vi "LaserMaster.vi"() -> ()   [LabVIEW 2014]
uses:
  Serial/Serial.lvclass
  <vilib>/Utility/file.llb/Write To Spreadsheet File (string).vi
panel:
  out "Discovery?":bool
  out "Humidity Threshold":dbl
  in  "Power (mW) 2":dbl format="%#.0f"
  out "SavePath":path
  out "Start time":timestamp
  out "Step":dbl
  out "State next step":string
  in  "stop":bool
  out "Query backup List":string[][](array[string])=[["?L", " 0\r"], ["?K", " 0\r"], ["?F", " 0\r"], ["?FH", " 2\r"], ["?SHUTTER", " 0\r"], ["?UF", " 0\r"], ["?PHLDC", " 1\r"], ["?PZTMC", " 0\r"], ["?PZTXC", " 2.24\r"], ["?PZTYC", " 2.14\r"], ["?PHLDP", " 0\r"], ["?PZTMP", " 0\r"], ["?PZTXP", " 2.58\r"], ["?PXTYP", "  Query Error:?PXTYP\r"], ["?PTRK", "  Query Error:?PTRK\r"], ["?MDLK", " 0\r"], ["?PP", " 0.80\r"], ["?TS", " 0\r"], ["?SM", " 1\r"], ["?HM", " 1\r"], ["?VW", " 850\r"], ["?STPRPOS", " 2096\r"], ["?C", " 0.00\r"], ["?D1C", " 0.08\r"], ["?D2C", " -0.43\r"], ["?BT", " 20.07\r"], ["?D1T", " 24.20\r"], ["?D2T", " 24.20\r"], ["?VT", " 20.72\r"], ["?LBOT", " 148.45\r"], ["?ET", " 39.01\r"], ["?D1ST", " 24.20\r"], ["?D2ST", " 24.20\r"], ["?VST", " 30.00\r"], ["?LBOST", " 148.41\r"], ["?EST", " 39.00\r"], ["?D1TD", " 500.12\r"], ["?D2TD", " 464.53\r"], ["?VD", " 0.00\r"], ["?LBOD", " 5358.08\r"], ["?ED", " 2152.46\r"], ["?D1HST", " 21.35\r"], ["?D2HST", " 21.48\r"], ["?LBOH", " 1\r"], ["?LRS", " 2\r"], ["?D1SS", " 1\r"], ["?D2SS", " 1\r"], ["?VSS", " 0\r"], ["?LBOSS", " 1\r"], ["?ESS", " 1\r"], ["?D1H", "  351.54\r"], ["?D2H", "  351.52\r"], ["?HH", " 37\r"], ["?D1V", " 0.19\r"], ["?D2V", " 0.18\r"], ["?SV", " 8.26,8.26,9.57\r"], ["?MB", "  Query Error:?MB\r"], ["?PI", " 2BC\r"], ["?BV", " 13.24\r"], ["?AMDLK", " 1\r"], ["?PZTS", "  Query Error:?PZTS\r"], ["?TMAX", " 1080\r"], ["?TMIN", " 680\r"], ["?ALIGN", " 0\r"], ["?ALIGNP", " 250\r"], ["?ALIGNW", " 730\r"], ["?LFP", " 0\r"], ["?PZTXCM", " 8.11\r"], ["?PZTXCP", " -10.30\r"], ["?PZTXPM", " 8.11\r"], ["?PZTXPP", " 3.06\r"], ["?PZTYCM", " 8.11\r"], ["?PZTYCP", " -14.28\r"], ["?PZTYPM", " 8.11\r"], ["?PZTYPP", " 11.74\r"], ["?RH", " 0\r"], ["?SN", " 9571\r"], ["?ST", " Standby\r"], ["?GDDCURVE", " 0\r"], ["?GDD", " 0\r"], ["?GDDCURVEN", " ZERO\r"], ["?CURVEN", " OUT OF RANGE\r"], ["?COMP", " 1\r"], ["?HMCOMP", " 1\r"], ["?GDDMAX", " 17333\r"], ["?GDDMIN", "0"]]
  out "Laser Info":i32
  out "Shutter off time":dbl
  out "Quiting":dbl
  out "Backuper state":string
  in  "Tab Control":T1(tab)
  out "Power 2":i32
  in  "Align 2":bool
  in  "Shutter 2":bool
  in  "Lock":bool
  in  "Auto":bool
  out "Baseplate Temp (C)":dbl(slide) scale=20.0..40.0
  in  "Dither hold":bool
  in  "Shutter":bool
  out "Laser Status":bool
  out "Power (mW)":dbl(knob) scale=0.0..5000.0
  out "Walking":bool
  out "Sleeping":bool
  out "ModeLocked":bool
  out "Backing up":bool
  in  "Wavelength":dbl=920.0
  in  "GDD":dbl
  in  "QUIT":bool
  out "Max":string
  in  "Align":bool
  in  "Def. Wavelength":dbl=920.0
  in  "Dither auto":dbl=120.0
  in  "Dither timer":dbl=5.0
  out "Faults":string
  in  "Home motor":bool
  in  "Optimize":bool
  in  "WV Walk":bool
  in  "Standby Time (min)":dbl=120.0
  in  "Sleep":bool
  in  "Backup":bool
  in  "Auto-Backup \nIdle Time (min)":dbl=30.0
  out "Operating Status":string
  out "Tunning Status":i32
  out "Idle Time":dbl format="%.1f"
  out "Laser On Time":dbl format="%#.1f"
  in  "Laser Control":bool
  in  "Command Line":string
  out "Laser Response":string
  in  "Refresh":bool
  out "Query List":string[][](array[string])
  out "queue #":i32
  # "LASER"
  # "LASER fine-tune"
  # "BACKUP"
  # "Timers"
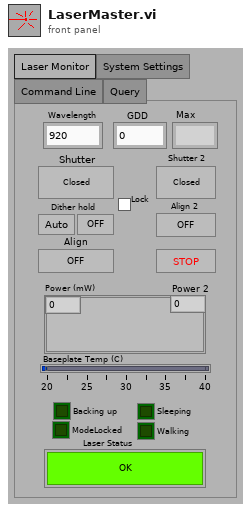
[diagram p1: front panel]
types:
  T1 = enum32{"Laser Monitor", "System Settings", "Command Line", "Query"}
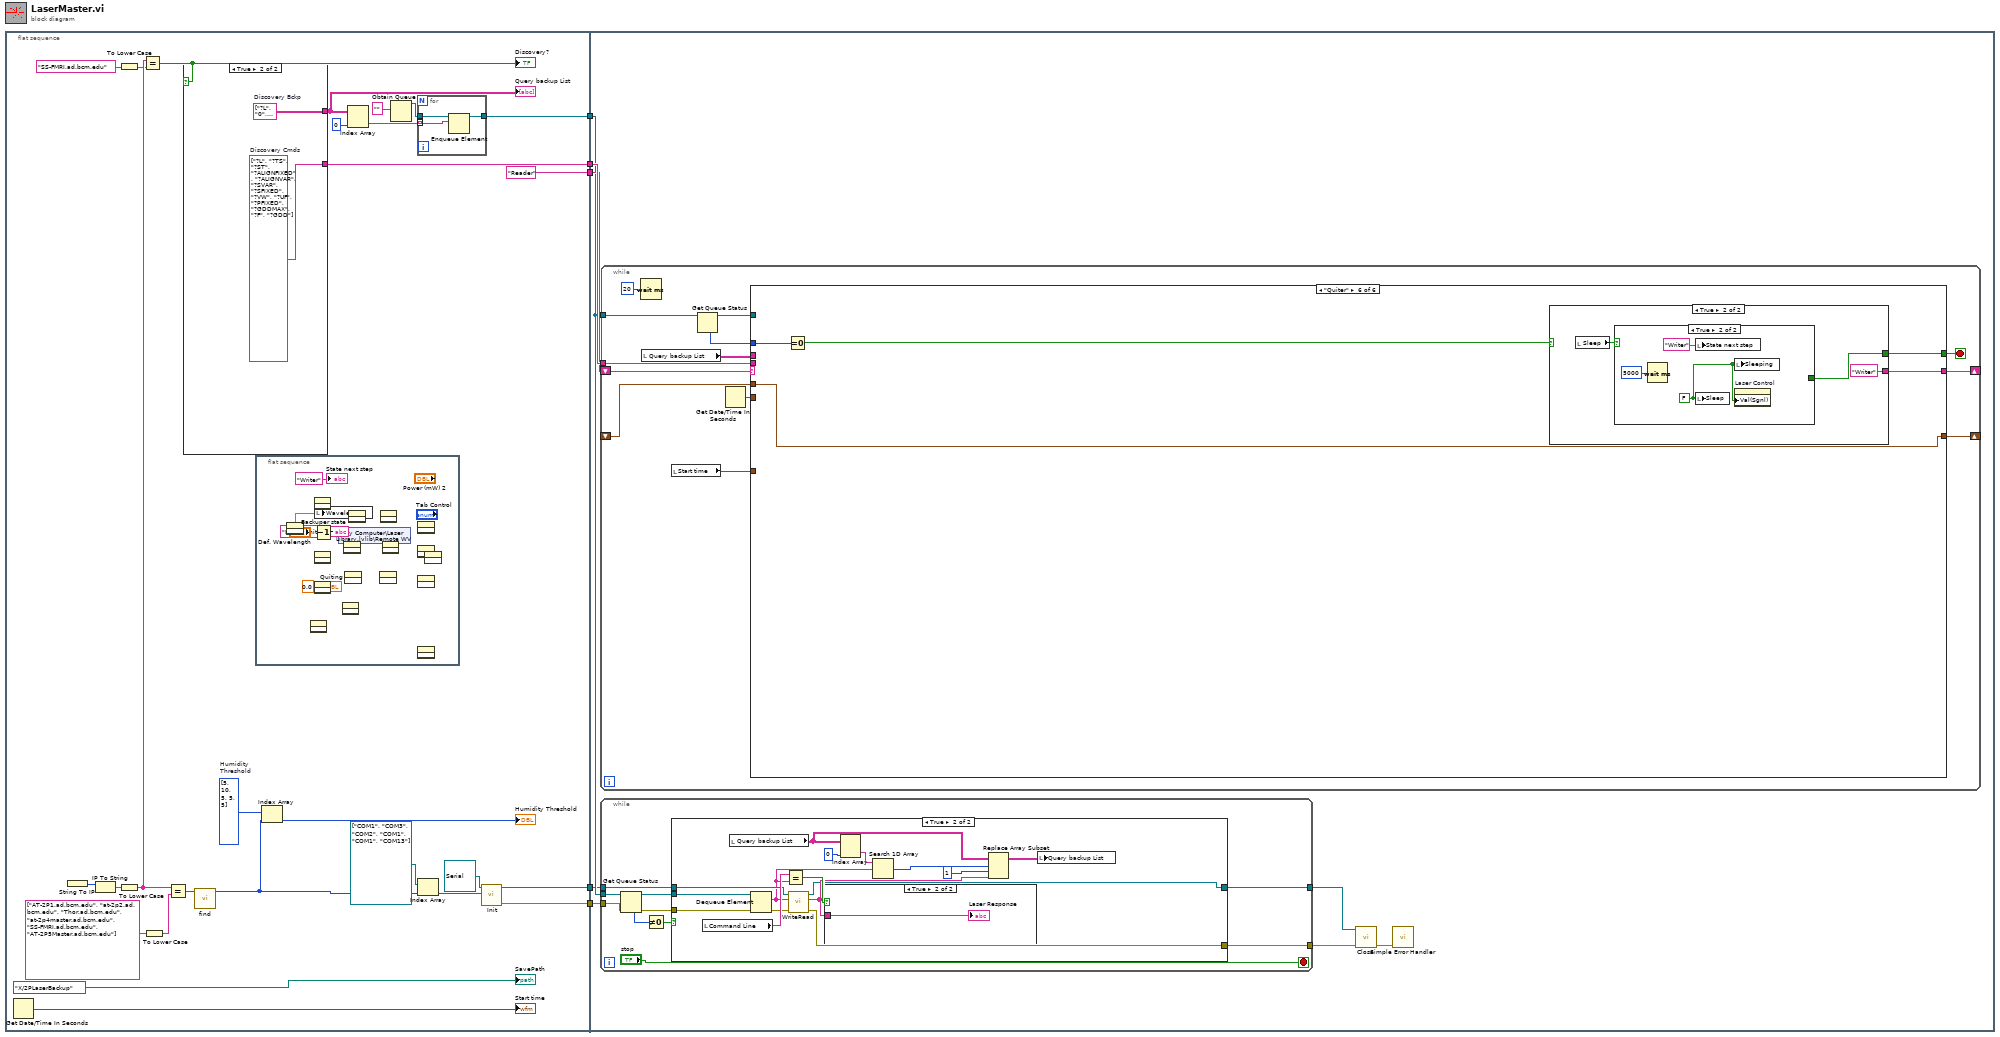
[diagram p0: block diagram]
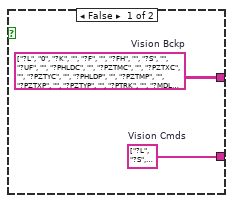
[diagram p2: hidden frame]
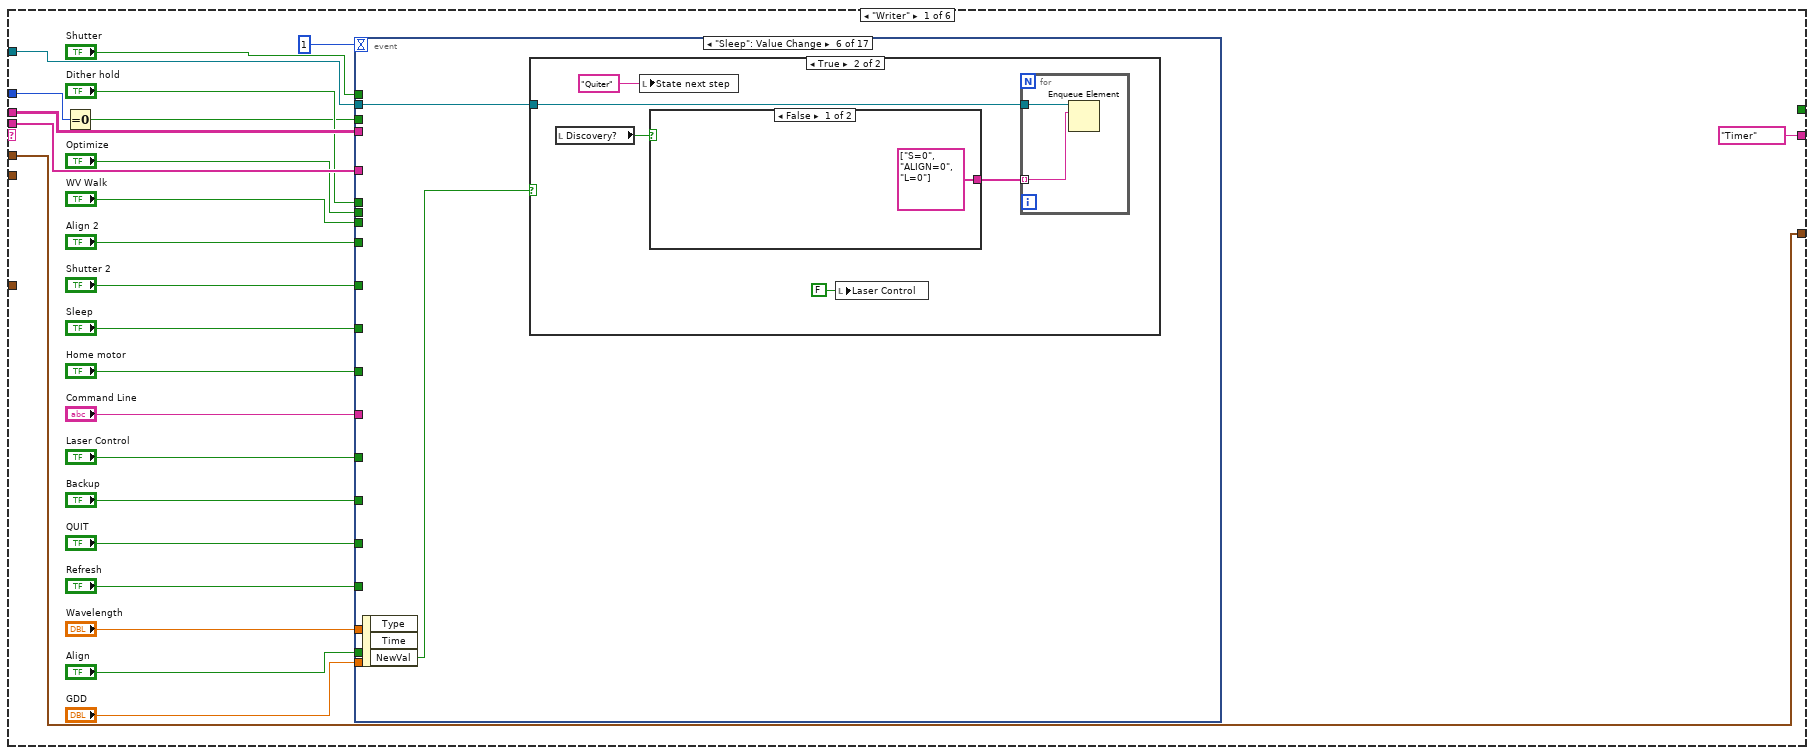
[diagram p5: hidden frame]
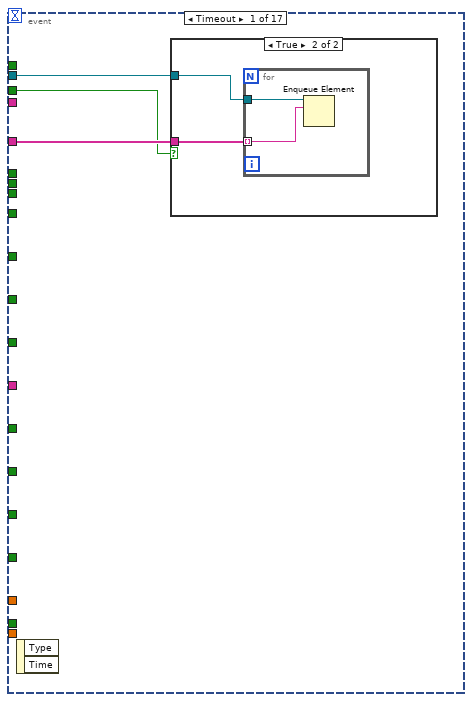
[diagram p6: hidden frame]
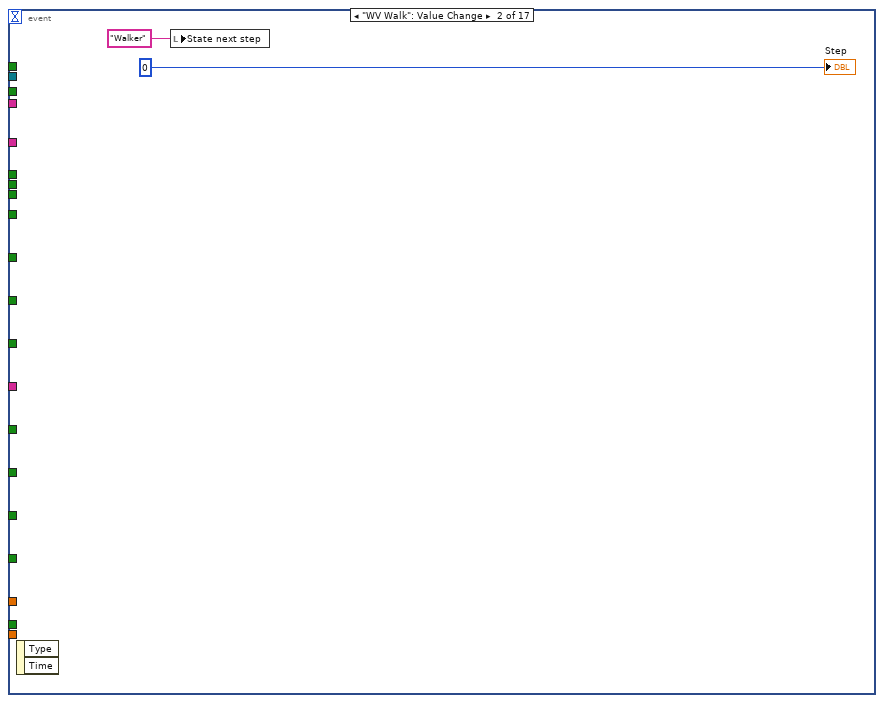
[diagram p8: hidden frame]
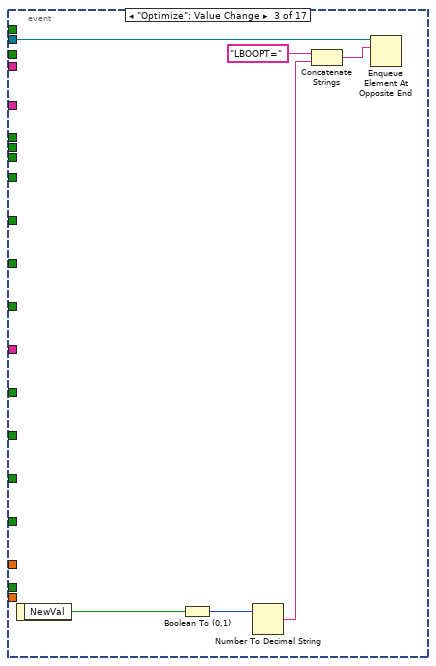
[diagram p9: hidden frame]
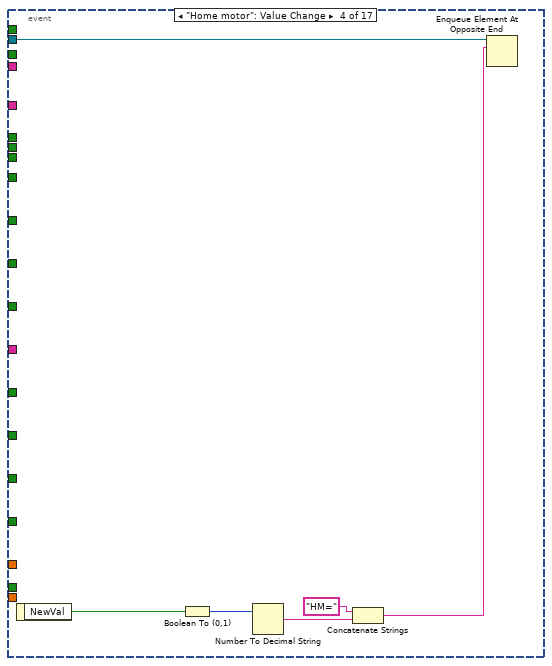
[diagram p10: hidden frame]
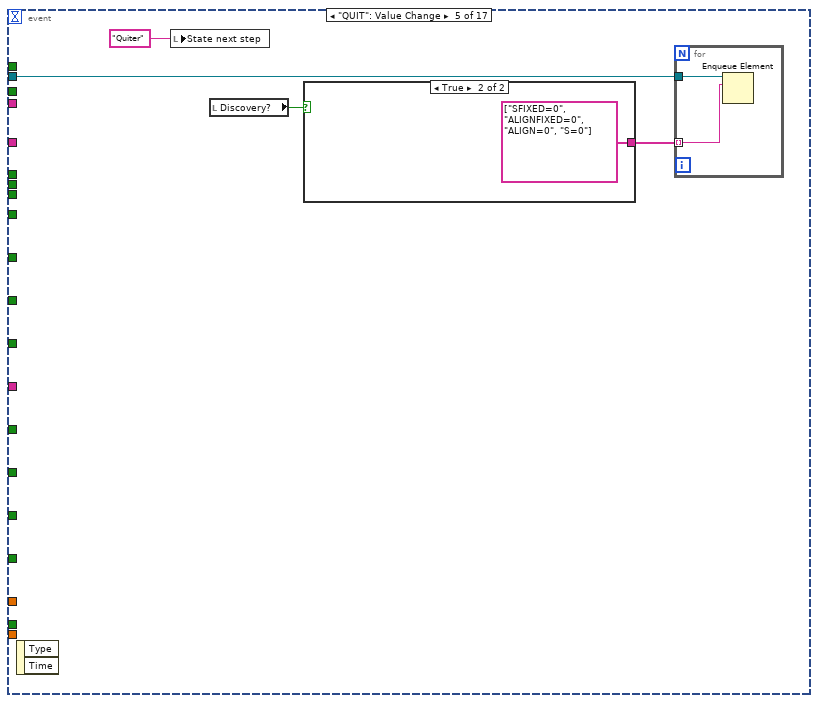
[diagram p11: hidden frame]
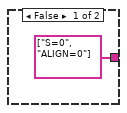
[diagram p12: hidden frame]
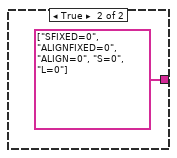
[diagram p14: hidden frame]
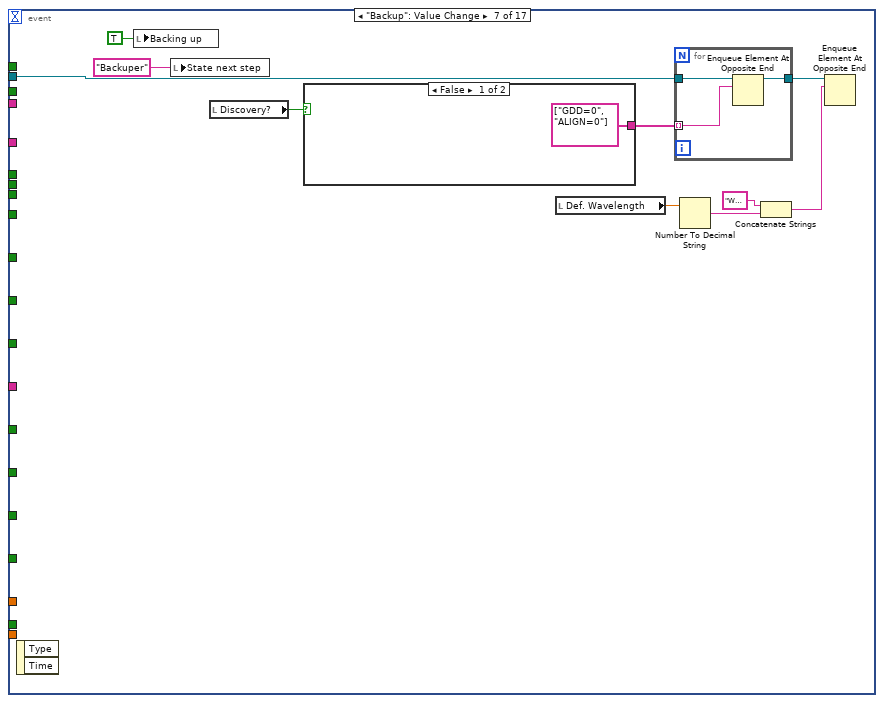
[diagram p15: hidden frame]
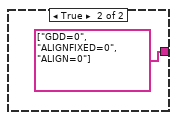
[diagram p16: hidden frame]
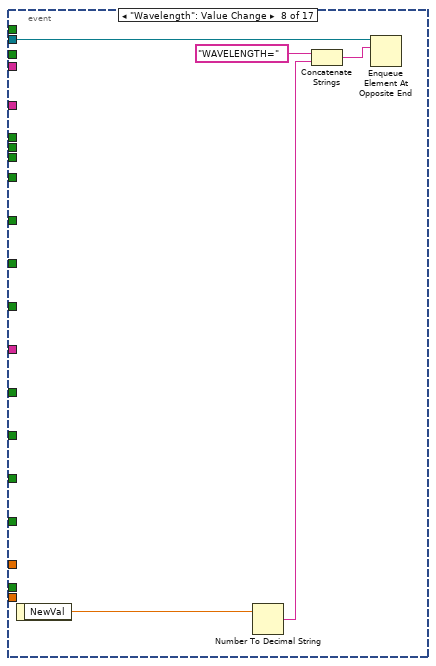
[diagram p17: hidden frame]
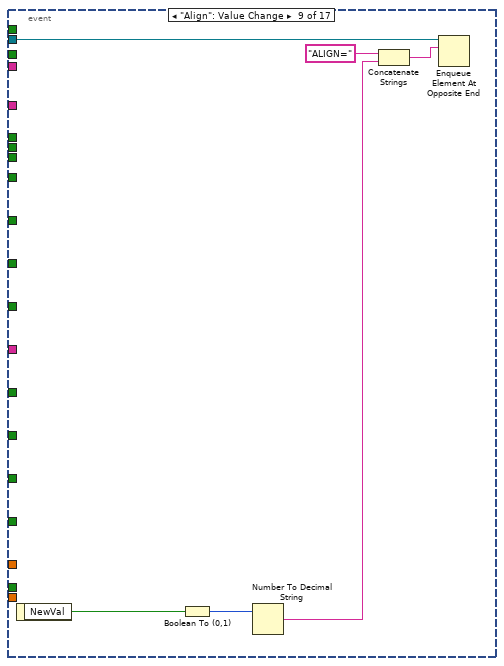
[diagram p18: hidden frame]
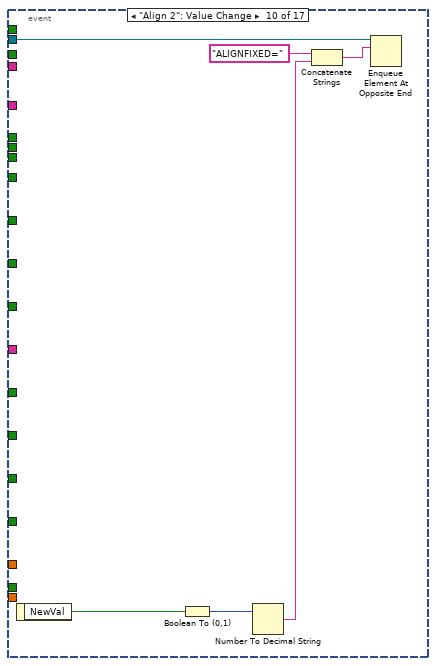
[diagram p19: hidden frame]
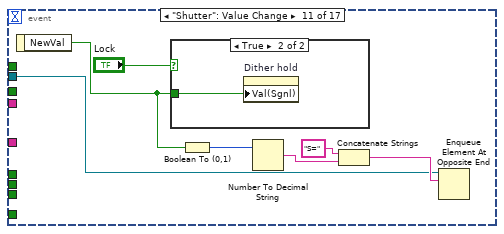
[diagram p20: hidden frame]
diagram:
  n1 = flat-sequence {
    tunnel: [w27] -> w5
    tunnel: [w10] -> w4
    tunnel: ["Reader"] -> w3
    tunnel: [w7] -> w2
    tunnel: [w6] -> w1
    tunnel: w5 -> [w50]
    tunnel: w4 -> [w52]
    tunnel: w3 -> [w51]
    tunnel: w2 -> [w49]
    tunnel: w1 -> [w48]
    frame #0 {
      w19 = i32[] [5, 10, 5, 5, 5]  # Humidity  Threshold
      n2 = Get Date/Time In Seconds() -> (seconds since 1Jan1904=→"Start time":timestamp)
      n3 = String To IP() -> (0:w24:u32)  [unwired: 1 in]
      n4 = IP To String(2:w24) -> (0:w22:string)  [unwired: 1 in]
      n5 = To Lower Case(string="SS-FMRI.ad.bcm.edu") -> (all lower case string=w13:string)
      n6 = To Lower Case(string=w22) -> (all lower case string=w15:string)
      n7 = Equal?(x=w15, y=w13) -> (x = y?=w12:bool)
      "Discovery?" <- w12
      n8 = To Lower Case(string=string[] ["AT-2P1.ad.bcm.edu", "at-2p2.ad.bcm.edu", "Thor.ad.bcm.edu", "at-2p4master.ad.bcm.edu", "SS-FMRI.ad.bcm.edu", "AT-2P5Master.ad.bcm.edu"]) -> (all lower case string=w23:string[])
      n9 = Equal?(x=w15, y=w23) -> (x = y?=w17:bool[])
      n10 = case shown="True" w12 {
        tunnel: [w34 w36] -> w11
        tunnel: [w33 w35] -> w10
        frame False {
          w33 = string[] ["?L", "?S", "?VW", "?ALIGN", "?PHLDP", "?UF", "?GDD", "?TS", "?ST", "?MDLK", "?GDDMAX", "?F", "?RH", "?BT"]  # Vision Cmds
          w34 = string[][] [["?L", "0"], ["?K", ""], ["?F", ""], ["?FH", ""], ["?S", ""], ["?UF", ""], ["?PHLDC", ""], ["?PZTMC", ""], ["?PZTXC", ""], ["?PZTYC", ""], ["?PHLDP", ""], ["?PZTMP", ""], ["?PZTXP", ""], ["?PZTYP", ""], ["?PTRK", ""], ["?MDLK", ""], ["?PP", ""], ["?TS", ""], ["?SM", ""], ["?HM", ""], ["?VW", ""], ["?STPRPOS", ""], ["?C", ""], ["?D1C", ""], ["?D2C", ""], ["?BT", ""], ["?D1T", ""], ["?D2T", ""], ["?VT", ""], ["?LBOT", ""], ["?ET", ""], ["?D1ST", ""], ["?D2ST", ""], ["?VST", ""], ["?LBOST", ""], ["?EST", ""], ["?D1TD", ""], ["?D2TD", ""], ["?VD", ""], ["?LBOD", ""], ["?ED", ""], ["?D1HST", ""], ["?D2HST", ""], ["?LBOH", ""], ["?LRS", ""], ["?D1SS", ""], ["?D2SS", ""], ["?VSS", ""], ["?LBOSS", ""], ["?ESS", ""], ["?D1H", ""], ["?D2H", ""], ["?HH", ""], ["?D1V", ""], ["?D2V", ""], ["?SV", ""], ["?PI", ""], ["?BV", ""], ["?AMDLK", ""], ["?PZTS", ""], ["?TMAX", ""], ["?TMIN", ""], ["?ALIGN", ""], ["?ALIGNP", ""], ["?ALIGNW", ""], ["?LFP", ""], ["?PZTXCM", ""], ["?PZTXCP", ""], ["?PZTXPM", ""], ["?PZTXPP", ""], ["?PZTYCM", ""], ["?PZTYCP", ""], ["?PZTYPM", ""], ["?PZTYPP", ""], ["?RH", ""], ["?SN", ""], ["?ST", ""], ["?GDDCURVE", ""], ["?GDD", ""], ["?GDDCURVEN", ""], ["?COMP", ""], ["?HMCOMP", ""], ["?GDDMAX", ""], ["?GDDMIN", ""]]  # Vision Bckp
        }
        frame True {
          w35 = string[] ["?L", "?TS", "?ST", "?ALIGNFIXED", "?ALIGNVAR", "?SVAR", "?SFIXED", "?VW", "?UF", "?PFIXED", "?GDDMAX", "?F", "?GDD"]  # Discovery Cmds
          w36 = string[][] [["?L", "0"], ["?K", ""], ["?TS", ""], ["?ST", ""], ["?ALIGNFIXED", ""], ["?ALIGNVAR", ""], ["?SVAR", ""], ["?SFIXED", ""], ["?VW", ""], ["?UF", ""], ["?PFIXED", ""], ["?HB", ""], ["?HRB", ""], ["?GDDCURVE", ""], ["?GDDCURVEN", ""], ["?GDD", ""], ["?GDDMAX", ""], ["?GDDMIN", ""], ["?SN", ""], ["?F", ""], ["?FT", ""], ["?FH", ""], ["?FHT", ""]]  # Discovery Bckp
        }
      }
      "Query backup List" <- w11
      n11 = call "find.vi"("Array"=w17) -> ("Index"=w16:i32)  [unwired: 10 in]
      n12 = flat-sequence {
        frame #0 {
          n13 = invoke on="ModeLocked" class="Bool (strict)" method="Reinit To Default"() -> ()  [unwired: 3 in, 3 out]
          n14 = invoke on="Align" class="Bool (strict)" method="Reinit To Default"() -> ()  [unwired: 3 in, 3 out]
          n15 = Decrement(x="Def. Wavelength") -> (x-1=w38:dbl)
          n16 = invoke on="Home motor" class="Bool" method="Reinit To Default"() -> ()  [unwired: 3 in, 3 out]
          n17 = invoke on="stop" class="Bool (strict)" method="Reinit To Default"() -> ()  [unwired: 3 in, 3 out]
          n18 = invoke on="Sleep" class="Bool (strict)" method="Reinit To Default"() -> ()  [unwired: 3 in, 3 out]
          n19 = local write "Wavelength"("Def. Wavelength") -> ()
          n20 = shared-variable "My Computer\\Laser Library.lvlib\\Remote WV"(w38) -> ()  [unwired: 1 in, 1 out]
          n21 = invoke on="WV Walk" class="Bool (strict)" method="Reinit To Default"() -> ()  [unwired: 3 in, 3 out]
          n22 = invoke on="Walking" class="Bool (strict)" method="Reinit To Default"() -> ()  [unwired: 3 in, 3 out]
          n23 = invoke on="Backup" class="Bool (strict)" method="Reinit To Default"() -> ()  [unwired: 3 in, 3 out]
          n24 = invoke on="Auto" class="Bool (strict)" method="Reinit To Default"() -> ()  [unwired: 3 in, 3 out]
          n25 = invoke on="Optimize" class="Bool" method="Reinit To Default"() -> ()  [unwired: 3 in, 3 out]
          n26 = invoke on="Sleeping" class="Bool (strict)" method="Reinit To Default"() -> ()  [unwired: 3 in, 3 out]
          n27 = invoke on="Refresh" class="Bool (strict)" method="Reinit To Default"() -> ()  [unwired: 3 in, 3 out]
          n28 = invoke on="Idle Time" class="DigNum (strict)" method="Reinit To Default"() -> ()  [unwired: 3 in, 3 out]
          n29 = invoke on="Laser Control" class="Bool (strict)" method="Reinit To Default"() -> ()  [unwired: 3 in, 3 out]
          n30 = invoke on="Dither hold" class="Bool (strict)" method="Reinit To Default"() -> ()  [unwired: 3 in, 3 out]
          n31 = invoke on="Backing up" class="Bool (strict)" method="Reinit To Default"() -> ()  [unwired: 3 in, 3 out]
          n32 = invoke on="QUIT" class="Bool (strict)" method="Reinit To Default"() -> ()  [unwired: 3 in, 3 out]
          "Backuper state" <- "BackupInit"
          "Quiting" <- 0.0 ("Quiting")
          "State next step" <- "Writer"
        }
      }
      n33 = Index Array(array=w19, index=w16) -> (element=→"Humidity Threshold":i32)
      n34 = Index Array(array=w11, index (col)=0 ("disabled index (col)")) -> (element=w29:string[])  [unwired: 1 in]
      n35 = Obtain Queue(element data type="") -> (queue out=w31:refnum<queue>)  [unwired: 4 in, 2 out]
      n36 = for {
        tunnel: w31 -> [w44]
        tunnel: w29 -> [w43] mode=indexing
        tunnel: [w42] -> w27
        n37 = Enqueue Element(queue=w44, element=w43) -> (queue out=w42:refnum<queue>)  [unwired: 2 in, 2 out]
      }
      n38 = Index Array(array=refnum<visa-resource-name>[] ["COM1", "COM3", "COM2", "COM1", "COM1", "COM13"], index=w16) -> (element=w9:refnum<visa-resource-name>)
      n39 = call-dynamic "Init.vi"("serial port"=w9, "Serial in"=refnum<class "Serial.lvclass"> refnum ("Serial.lvclass")) -> ("error out"=w6:errorcluster, "Serial out"=w7:refnum<class "Serial.lvclass">)  [unwired: 8 in]
      "SavePath" <- path "X:/2PLaserBackup"
    }
    frame #1 {
      n40 = while {
        tunnel: w50 -> [w91]
        tunnel: w52 -> [w92]
        shift-right: [w93] -> _
        shift-left: w51 -> [w94]
        shift-right: [w83] -> _
        shift-left: _ -> [w82]
        stop <- w88 stop-if-true
        n41 = Wait (ms)(milliseconds to wait=u32 20) -> ()  [unwired: 1 out]
        n42 = local read "Query backup List"() -> (w90:string[][])
        n43 = local read "Start time"() -> (w84:timestamp)
        n44 = Get Queue Status(queue=w91) -> (queue out=w87:refnum<queue>, # elements in queue=w86:i32)  [unwired: 2 in, 6 out]
        n45 = Get Date/Time In Seconds() -> (seconds since 1Jan1904=w85:timestamp)
        n46 = case shown="\"Quiter\"" w94 {
          tunnel: w87 -> [w118 _ w301 _ _ _]
          tunnel: w90 -> [w117 _ w305 _ w501 _]
          tunnel: w92 -> [w116 _ w306 _ _ _]
          tunnel: ["Timer" "Interpreter" w304 "Writer" "Writer" w527] -> w93
          tunnel: w86 -> [w115 _ w303 _ _ w529]
          tunnel: [_ _ _ _ _ w526] -> w88
          tunnel: w85 -> [_ w235 _ _ _ _]
          tunnel: w84 -> [_ w239 _ _ _ _]
          tunnel: [w97 w236 w302 w483 w498 w525] -> w83
          tunnel: w82 -> [w97 w234 w302 w483 w498 w525]
          frame "Writer" {
            n47 = Equal To 0?(x=w115) -> (x = 0?=w103:bool)
            n48 = event shown="[5] \"Sleep\": Value Change" {
              selector: _ -> [_ _ _ _ _ _ _ _ _ _ _ _ _ _ _ _ _]
              dyn-events: _ -> [_ _ _ _ _ _ _ _ _ _ _ _ _ _ _ _ _]
              timeout: 1 -> [_ _ _ _ _ _ _ _ _ _ _ _ _ _ _ _ _]
              tunnel: w118 -> [w121 _ w128 w135 w143 w149 w168 w175 w180 w186 w193 w200 w206 w213 w218 w225 w227]
              tunnel: "Shutter" -> [_ _ _ _ _ _ _ _ _ _ _ _ _ _ _ _ _]
              tunnel: "Dither hold" -> [_ _ _ _ _ _ _ _ _ _ _ _ _ _ _ _ _]
              tunnel: "GDD" -> [_ _ _ _ _ _ _ _ _ _ _ _ _ _ _ _ _]
              tunnel: "Align" -> [_ _ _ _ _ _ _ _ _ _ _ _ _ _ _ _ _]
              tunnel: "Wavelength" -> [_ _ _ _ _ _ _ _ _ _ _ _ _ _ _ _ _]
              tunnel: "Laser Control" -> [_ _ _ _ _ _ _ _ _ _ _ _ _ _ _ _ _]
              tunnel: "Command Line" -> [_ _ _ _ _ _ _ _ _ _ _ _ _ _ _ _ _]
              tunnel: w117 -> [_ _ _ _ _ _ _ _ _ _ _ _ w205 _ _ _ _]
              tunnel: "Refresh" -> [_ _ _ _ _ _ _ _ _ _ _ _ _ _ _ _ _]
              tunnel: w116 -> [w120 _ _ _ _ _ _ _ _ _ _ _ _ _ _ _ _]
              tunnel: "QUIT" -> [_ _ _ _ _ _ _ _ _ _ _ _ _ _ _ _ _]
              tunnel: "Backup" -> [_ _ _ _ _ _ _ _ _ _ _ _ _ _ _ _ _]
              tunnel: w103 -> [w119 _ _ _ _ _ _ _ _ _ _ _ _ _ _ _ _]
              tunnel: "WV Walk" -> [_ _ _ _ _ _ _ _ _ _ _ _ _ _ _ _ _]
              tunnel: "Optimize" -> [_ _ _ _ _ _ _ _ _ _ _ _ _ _ _ _ _]
              tunnel: "Home motor" -> [_ _ _ _ _ _ _ _ _ _ _ _ _ _ _ _ _]
              tunnel: "Sleep" -> [_ _ _ _ _ _ _ _ _ _ _ _ _ _ _ _ _]
              tunnel: "Shutter 2" -> [_ _ _ _ _ _ _ _ _ _ _ _ _ _ _ _ _]
              tunnel: "Align 2" -> [_ _ _ _ _ _ _ _ _ _ _ _ _ _ _ _ _]
              event Timeout {
                n49 = event-data() -> ()  [unwired: 1 in, 2 out]
                n50 = case shown="True" w119 {
                  tunnel: w121 -> [_ w123]
                  tunnel: w120 -> [_ w122]
                  frame False {
                  }
                  frame True {
                    n51 = for {
                      tunnel: w123 -> [w125]
                      tunnel: w122 -> [w124] mode=indexing
                      n52 = Enqueue Element(queue=w125, element=w124) -> ()  [unwired: 2 in, 3 out]
                    }
                  }
                }
              }
              event "WV Walk": Value Change {
                n53 = event-data() -> ()  [unwired: 1 in, 2 out]
                n54 = local write "State next step"("Walker") -> ()
                "Step" <- 0
              }
              event "Optimize": Value Change {
                n55 = event-data() -> ("NewVal"=w129:bool)  [unwired: 1 in]
                n56 = Boolean To (0,1)(Boolean=w129) -> (0, 1=w132:i16)
                n57 = Number To Decimal String(number=w132) -> (decimal integer string=w133:string)  [unwired: 1 in]
                n58 = Concatenate Strings("LBOOPT=", w133) -> (w130:string)
                n59 = Enqueue Element At Opposite End(queue=w128, element=w130) -> ()  [unwired: 2 in, 3 out]
              }
              event "Home motor": Value Change {
                n60 = event-data() -> ("NewVal"=w134:bool)  [unwired: 1 in]
                n61 = Boolean To (0,1)(Boolean=w134) -> (0, 1=w138:i16)
                n62 = Number To Decimal String(number=w138) -> (decimal integer string=w139:string)  [unwired: 1 in]
                n63 = Concatenate Strings("HM=", w139) -> (w136:string)
                n64 = Enqueue Element At Opposite End(queue=w135, element=w136) -> ()  [unwired: 2 in, 3 out]
              }
              event "QUIT": Value Change {
                n65 = event-data() -> ()  [unwired: 1 in, 2 out]
                n66 = local write "State next step"("Quiter") -> ()
                n67 = local read "Discovery?"() -> (w140:bool)
                n68 = case shown="True" w140 {
                  tunnel: [string[] ["S=0", "ALIGN=0"] string[] ["SFIXED=0", "ALIGNFIXED=0", "ALIGN=0", "S=0"]] -> w141
                  frame False {
                  }
                  frame True {
                  }
                }
                n69 = for {
                  tunnel: w143 -> [w147]
                  tunnel: w141 -> [w146] mode=indexing
                  n70 = Enqueue Element(queue=w147, element=w146) -> ()  [unwired: 2 in, 3 out]
                }
              }
              event "Sleep": Value Change {
                n71 = event-data() -> ("NewVal"=w148:bool)  [unwired: 1 in, 2 out]
                n72 = case shown="True" w148 {
                  tunnel: w149 -> [_ w153]
                  frame False {
                  }
                  frame True {
                    n73 = local read "Discovery?"() -> (w152:bool)
                    n74 = local write "State next step"("Quiter") -> ()
                    n75 = case shown="False" w152 {
                      tunnel: [string[] ["S=0", "ALIGN=0", "L=0"] string[] ["SFIXED=0", "ALIGNFIXED=0", "ALIGN=0", "S=0", "L=0"]] -> w151
                      frame False {
                      }
                      frame True {
                      }
                    }
                    n76 = local write "Laser Control"(FALSE ("Laser Control")) -> ()
                    n77 = for {
                      tunnel: w153 -> [w158]
                      tunnel: w151 -> [w157] mode=indexing
                      n78 = Enqueue Element(queue=w158, element=w157) -> ()  [unwired: 2 in, 3 out]
                    }
                  }
                }
              }
              event "Backup": Value Change {
                n79 = event-data() -> ()  [unwired: 1 in, 2 out]
                n80 = local write "Backing up"(TRUE ("Backing up ...")) -> ()
                n81 = local write "State next step"("Backuper") -> ()
                n82 = local read "Discovery?"() -> (w160:bool)
                n83 = case shown="False" w160 {
                  tunnel: [string[] ["GDD=0", "ALIGN=0"] string[] ["GDD=0", "ALIGNFIXED=0", "ALIGN=0"]] -> w159
                  frame False {
                  }
                  frame True {
                  }
                }
                n84 = local read "Def. Wavelength"() -> (w164:dbl)
                n85 = for {
                  tunnel: w159 -> [w173] mode=indexing
                  tunnel: w168 -> [w172]
                  tunnel: [w171] -> w165
                  n86 = Enqueue Element At Opposite End(queue=w172, element=w173) -> (queue out=w171:refnum<queue>)  [unwired: 2 in, 2 out]
                }
                n87 = Number To Decimal String(number=w164) -> (decimal integer string=w162:string)  [unwired: 1 in]
                n88 = Concatenate Strings("WAVELENGTH=", w162) -> (w161:string)
                n89 = Enqueue Element At Opposite End(queue=w165, element=w161) -> ()  [unwired: 2 in, 3 out]
              }
              event "Wavelength": Value Change {
                n90 = event-data() -> ("NewVal"=w174:dbl)  [unwired: 1 in]
                n91 = Number To Decimal String(number=w174) -> (decimal integer string=w177:string)  [unwired: 1 in]
                n92 = Concatenate Strings("WAVELENGTH=", w177) -> (w178:string)
                n93 = Enqueue Element At Opposite End(queue=w175, element=w178) -> ()  [unwired: 2 in, 3 out]
              }
              event "Align": Value Change {
                n94 = event-data() -> ("NewVal"=w179:bool)  [unwired: 1 in]
                n95 = Boolean To (0,1)(Boolean=w179) -> (0, 1=w183:i16)
                n96 = Number To Decimal String(number=w183) -> (decimal integer string=w184:string)  [unwired: 1 in]
                n97 = Concatenate Strings("ALIGN=", w184) -> (w181:string)
                n98 = Enqueue Element At Opposite End(queue=w180, element=w181) -> ()  [unwired: 2 in, 3 out]
              }
              event "Align 2": Value Change {
                n99 = event-data() -> ("NewVal"=w185:bool)  [unwired: 1 in]
                n100 = Boolean To (0,1)(Boolean=w185) -> (0, 1=w189:i16)
                n101 = Number To Decimal String(number=w189) -> (decimal integer string=w190:string)  [unwired: 1 in]
                n102 = Concatenate Strings("ALIGNFIXED=", w190) -> (w187:string)
                n103 = Enqueue Element At Opposite End(queue=w186, element=w187) -> ()  [unwired: 2 in, 3 out]
              }
              event "Shutter": Value Change {
                n104 = event-data() -> ("NewVal"=w191:bool)  [unwired: 1 in]
                n105 = case shown="True" "Lock" {
                  tunnel: w191 -> [_ w198]
                  frame False {
                  }
                  frame True {
                    n106 = property on="Dither hold" class="Bool (strict)"("Val(Sgnl)"=w198) -> ()  [unwired: 2 in, 2 out]
                  }
                }
                n107 = Boolean To (0,1)(Boolean=w191) -> (0, 1=w196:i16)
                n108 = Number To Decimal String(number=w196) -> (decimal integer string=w197:string)  [unwired: 1 in]
                n109 = Concatenate Strings("S=", w197) -> (w194:string)
                n110 = Enqueue Element At Opposite End(queue=w193, element=w194) -> ()  [unwired: 2 in, 3 out]
              }
              event "Shutter 2": Value Change {
                n111 = event-data() -> ("NewVal"=w199:bool)  [unwired: 1 in]
                n112 = Boolean To (0,1)(Boolean=w199) -> (0, 1=w203:i16)
                n113 = Number To Decimal String(number=w203) -> (decimal integer string=w204:string)  [unwired: 1 in]
                n114 = Concatenate Strings("SFIXED=", w204) -> (w201:string)
                n115 = Enqueue Element At Opposite End(queue=w200, element=w201) -> ()  [unwired: 2 in, 3 out]
              }
              event "Refresh": Value Change {
                n116 = event-data() -> ()  [unwired: 1 in, 1 out]
                n117 = local write "Refresh"(FALSE ("Backup")) -> ()
                n118 = Index Array(array=w205, index (col)=0 ("disabled index (col)")) -> (element=w208:string[])  [unwired: 1 in]
                n119 = for {
                  tunnel: w206 -> [w211]
                  tunnel: w208 -> [w210] mode=indexing
                  n120 = Enqueue Element(queue=w211, element=w210) -> ()  [unwired: 2 in, 3 out]
                }
              }
              event "Dither hold": Value Change {
                n121 = event-data() -> ("NewVal"=w212:bool)  [unwired: 1 in]
                n122 = Boolean To (0,1)(Boolean=w212) -> (0, 1=w216:i16)
                n123 = Number To Decimal String(number=w216) -> (decimal integer string=w217:string)  [unwired: 1 in]
                n124 = Concatenate Strings("PHLDP=", w217) -> (w214:string)
                n125 = Enqueue Element At Opposite End(queue=w213, element=w214) -> ()  [unwired: 2 in, 3 out]
              }
              event "Laser Control": Value Change {
                n126 = event-data() -> ("NewVal"=w219:bool)  [unwired: 1 in]
                n127 = Boolean To (0,1)(Boolean=w219) -> (0, 1=w222:i16)
                n128 = Number To Decimal String(number=w222) -> (decimal integer string=w223:string)  [unwired: 1 in]
                n129 = Concatenate Strings("L=", w223) -> (w220:string)
                n130 = Enqueue Element At Opposite End(queue=w218, element=w220) -> ()  [unwired: 2 in, 3 out]
              }
              event "Command Line": Value Change {
                n131 = event-data() -> ("NewVal"=w224:string)  [unwired: 1 in]
                n132 = Enqueue Element At Opposite End(queue=w225, element=w224) -> ()  [unwired: 2 in, 3 out]
              }
              event "GDD": Value Change {
                n133 = event-data() -> ("NewVal"=w226:dbl)  [unwired: 1 in]
                n134 = Number To Decimal String(number=w226) -> (decimal integer string=w229:string)  [unwired: 1 in]
                n135 = Concatenate Strings("GDD=", w229) -> (w230:string)
                n136 = Enqueue Element At Opposite End(queue=w227, element=w230) -> ()  [unwired: 2 in, 3 out]
              }
            }
          }
          frame "Timer" {
            n137 = Subtract(x=w235, y=w239) -> (x-y=w242:dbl)
            n138 = local read "Tunning Status"() -> (w259:i32)
            n139 = local read "Laser Control"() -> (w258:bool)
            n140 = local read "Power (mW)"() -> (w232:dbl)
            n141 = case shown="True" "Auto" {
              tunnel: w235 -> [w261 w268]
              tunnel: [w261 w267] -> w236
              tunnel: w234 -> [_ w266]
              frame False {
              }
              frame True {
                n142 = Subtract(x=w268, y=w266) -> (x-y=w270:dbl)
                n143 = local read "Dither hold"() -> (w262:bool)
                n144 = Select(t="Dither auto", s=w262, f="Dither timer") -> (s? t:f=w263:dbl)
                n145 = Greater?(x=w270, y=w263) -> (0:w269:bool)
                n146 = case shown="True" w269 {
                  tunnel: w268 -> [_ w274]
                  tunnel: [w271 w274] -> w267
                  tunnel: w266 -> [w271 _]
                  tunnel: w262 -> [_ w273]
                  frame False {
                  }
                  frame True {
                    n147 = Not(x=w273) -> (.not. x?=w272:bool)
                    n148 = property on="Dither hold" class="Bool (strict)"("Val(Sgnl)"=w272) -> ()  [unwired: 2 in, 2 out]
                  }
                }
              }
            }
            n149 = Not(x=w258) -> (.not. x?=w254:bool)
            n150 = Equal To 0?(x=w259) -> (x = 0?=w253:bool)
            n151 = Less?(x=w232, y=1.0) -> (x < y?=w231:bool)
            n152 = local read "Shutter off time"() -> (w249:dbl)
            n153 = local read "Shutter"() -> (w250:bool)
            n154 = Compound Arithmetic op=AND(w231, w254, w253) -> (w255:bool)
            n155 = Divide(x=w242, y=60.0 ("x")) -> (x/y=w240:dbl)
            n156 = case shown="False" w255 {
              tunnel: [w275 w286] -> w252
              tunnel: [w279 w286] -> w251
              tunnel: w250 -> [w278 _]
              tunnel: w249 -> [w277 _]
              tunnel: [w276 w286] -> w248
              tunnel: w240 -> [w275 _]
              frame False {
                n157 = case shown="False" w278 {
                  tunnel: [w282 0] -> w279
                  tunnel: w275 -> [w281 w283]
                  tunnel: w277 -> [w280 _]
                  tunnel: [w280 w283] -> w276
                  frame False {
                    n158 = Subtract(x=w281, y=w280) -> (x-y=w282:dbl)
                  }
                  frame True {
                  }
                }
              }
              frame True {
                w286 = 0
                n159 = Get Date/Time In Seconds() -> (seconds since 1Jan1904=w285:timestamp)
                n160 = local write "Start time"(w285) -> ()
              }
            }
            "Laser On Time" <- w252
            "Idle Time" <- w251
            "Shutter off time" <- w248
            n161 = local read "Backing up"() -> (w243:bool)
            n162 = Greater?(x=w251, y="Auto-Backup \nIdle Time (min)") -> (0:w246:bool)
            n163 = Greater?(x=w251, y="Standby Time (min)") -> (0:w238:bool)
            n164 = Not(x=w243) -> (.not. x?=w245:bool)
            n165 = case shown="True" w238 {
              tunnel: [FALSE ("Sleeping") w288] -> w247
              frame False {
              }
              frame True {
                w288 = TRUE
                n166 = property on="Sleep" class="Bool (strict)"("Val(Sgnl)"=w288) -> ()  [unwired: 2 in, 2 out]
              }
            }
            "Sleeping" <- w247
            n167 = And(x=w246, y=w245) -> (x .and. y?=w244:bool)
            n168 = case shown="True" w244 {
              frame False {
              }
              frame True {
                n169 = Get Date/Time In Seconds() -> (seconds since 1Jan1904=w295:timestamp)
                n170 = Format Date/Time String(time format string (%c)="%Y-%m-%d-*", seconds (now)=w295) -> (date/time string=w292:string)  [unwired: 1 in]
                n171 = String To IP() -> (0:w293:u32)  [unwired: 1 in]
                n172 = local read "SavePath"() -> (w289:path)
                n173 = IP To String(2:w293) -> (0:w290:string)  [unwired: 1 in]
                n174 = Concatenate Strings(w292, ".csv" ("string")) -> (w297:string)
                n175 = call "create unique folder.vi"("string"=w290, "path 2"=w289) -> ("path"=w298:path)  [unwired: 9 in]
                n176 = call <vilib>:"Recursive File List.vi"("pattern"=w297, "Folder Path"=w298) -> ("Number of Files"=w299:i32)  [unwired: 5 in, 4 out]
                n177 = Equal To 0?(x=w299) -> (x = 0?=w291:bool)
                n178 = case shown="True" w291 {
                  frame False {
                  }
                  frame True {
                    n179 = property on="Backup" class="Bool (strict)"("Val(Sgnl)"=TRUE) -> ()  [unwired: 2 in, 2 out]
                  }
                }
              }
            }
          }
          frame "Interpreter", Default {
            n180 = stacked-sequence {
              tunnel: w306 -> [_ w321 _ _ _]
              tunnel: w305 -> [_ w320 _ w448 _]
              tunnel: w301 -> [w307 _ _ _ _]
              frame #0 {
                n181 = local read "Command Line"() -> (w309:string)
                n182 = feedback-in #1(w309) -> ()
                n183 = feedback #1() -> (w310:string)  [unwired: 1 in]
                n184 = Not Equal?(x=w310, y=w309) -> (x != y?=w308:bool)
                n185 = case shown="False" w308 {
                  tunnel: w307 -> [_ w312]
                  tunnel: w309 -> [_ w311]
                  frame False {
                  }
                  frame True {
                    n186 = Enqueue Element At Opposite End(queue=w312, element=w311) -> ()  [unwired: 2 in, 3 out]
                  }
                }
              }
              frame #1 {
                n187 = local read "Faults"() -> (w314:string)
                n188 = for {
                  tunnel: w321 -> [w323] mode=indexing
                  tunnel: w320 -> [w324]
                  n189 = Index Array(array=w324, index (col)=0 ("disabled index (col)")) -> (element=w327:string[])  [unwired: 1 in]
                  n190 = Search 1D Array(1D array=w327, element=w323) -> (index of element=w325:i32)  [unwired: 1 in]
                  n191 = Index Array(array=w324, index (row)=w325, index (col)=1 ("disabled index (col)")) -> (element=w322:string)
                  n192 = case shown="\"?L\"" w323 {
                    tunnel: w322 -> [_ w332 w338 w343 w348 w356 w364 w372 w380 w384 w393 w396 w398 w406 w408 w410 w412 w413 w424 w426]
                    frame "False", Default {
                    }
                    frame "?L" {
                      n193 = Decimal String To Number(string=w332) -> (number=w329:i32)  [unwired: 2 in, 1 out]
                      n194 = String Length(string=w332) -> (length=w331:i32)
                      n195 = Equal To 0?(x=w331) -> (x = 0?=w330:bool)
                      n196 = case shown="False" w330 {
                        tunnel: w329 -> [w333 _]
                        frame False {
                          "Laser Info" <- w333
                        }
                        frame True {
                        }
                      }
                    }
                    frame "?S" {
                      n197 = Decimal String To Number(string=w338) -> (number=w339:i32)  [unwired: 2 in, 1 out]
                      n198 = local read "Shutter"() -> (w341:bool)
                      n199 = Not Equal To 0?(x=w339) -> (x != 0?=w340:bool)
                      n200 = And(x=w340, y=w341) -> (x .and. y?=w334:bool)
                      n201 = Select(t=cluster{u32, u32}[] [{12369084, 12369084}, {6618880, 6618880}] ("Colors [4]"), s=w334, f=cluster{u32, u32}[] [{12369084, 12369084}, {12369084, 12369084}] ("Colors [4]")) -> (s? t:f=w335:cluster{u32, u32}[])
                      n202 = property on="Shutter" class="Bool (strict)"("Colors [4]"=w335) -> ()  [unwired: 2 in, 2 out]
                    }
                    frame "?VW" {
                      n203 = Decimal String To Number(string=w343) -> (number=w342:i32)  [unwired: 2 in, 1 out]
                      n204 = property on="Wavelength" class="DigNum (strict)"("Value"=w342) -> ()  [unwired: 2 in, 2 out]
                      n205 = shared-variable ".\\Laser Library.lvlib\\WV"(w342) -> ()  [unwired: 1 in, 1 out]
                    }
                    frame "?SVAR" {
                      n206 = Decimal String To Number(string=w348) -> (number=w349:i32)  [unwired: 2 in, 1 out]
                      n207 = local read "Shutter"() -> (w351:bool)
                      n208 = Not Equal To 0?(x=w349) -> (x != 0?=w350:bool)
                      n209 = And(x=w350, y=w351) -> (x .and. y?=w344:bool)
                      n210 = Select(t=cluster{u32, u32}[] [{12369084, 12369084}, {6618880, 6618880}] ("Colors [4]"), s=w344, f=cluster{u32, u32}[] [{12369084, 12369084}, {12369084, 12369084}] ("Colors [4]")) -> (s? t:f=w345:cluster{u32, u32}[])
                      n211 = property on="Shutter" class="Bool (strict)"("Colors [4]"=w345) -> ()  [unwired: 2 in, 2 out]
                    }
                    frame "?SFIXED" {
                      n212 = Decimal String To Number(string=w356) -> (number=w357:i32)  [unwired: 2 in, 1 out]
                      n213 = local read "Shutter 2"() -> (w359:bool)
                      n214 = Not Equal To 0?(x=w357) -> (x != 0?=w358:bool)
                      n215 = And(x=w358, y=w359) -> (x .and. y?=w352:bool)
                      n216 = Select(t=cluster{u32, u32}[] [{12369084, 12369084}, {6618880, 6618880}] ("Colors [4]"), s=w352, f=cluster{u32, u32}[] [{12369084, 12369084}, {12369084, 12369084}] ("Colors [4]")) -> (s? t:f=w355:cluster{u32, u32}[])
                      n217 = property on="Shutter 2" class="Bool (strict)"("Colors [4]"=w355) -> ()  [unwired: 2 in, 2 out]
                    }
                    frame "?ALIGN" {
                      n218 = Decimal String To Number(string=w364) -> (number=w365:i32)  [unwired: 2 in, 1 out]
                      n219 = Not Equal To 0?(x=w365) -> (x != 0?=w367:bool)
                      n220 = local read "Align"() -> (w366:bool)
                      n221 = And(x=w367, y=w366) -> (x .and. y?=w361:bool)
                      n222 = Select(t=cluster{u32, u32}[] [{12369084, 12369084}, {6618880, 6618880}] ("Colors [4]"), s=w361, f=cluster{u32, u32}[] [{12369084, 12369084}, {12369084, 12369084}] ("Colors [4]")) -> (s? t:f=w360:cluster{u32, u32}[])
                      n223 = property on="Align" class="Bool (strict)"("Colors [4]"=w360) -> ()  [unwired: 2 in, 2 out]
                    }
                    frame "?ALIGNVAR" {
                      n224 = Decimal String To Number(string=w372) -> (number=w373:i32)  [unwired: 2 in, 1 out]
                      n225 = Not Equal To 0?(x=w373) -> (x != 0?=w375:bool)
                      n226 = local read "Align"() -> (w374:bool)
                      n227 = And(x=w375, y=w374) -> (x .and. y?=w368:bool)
                      n228 = Select(t=cluster{u32, u32}[] [{12369084, 12369084}, {6618880, 6618880}] ("Colors [4]"), s=w368, f=cluster{u32, u32}[] [{12369084, 12369084}, {12369084, 12369084}] ("Colors [4]")) -> (s? t:f=w369:cluster{u32, u32}[])
                      n229 = property on="Align" class="Bool (strict)"("Colors [4]"=w369) -> ()  [unwired: 2 in, 2 out]
                    }
                    frame "?ALIGNFIXED" {
                      n230 = Decimal String To Number(string=w380) -> (number=w381:i32)  [unwired: 2 in, 1 out]
                      n231 = local read "Align 2"() -> (w382:bool)
                      n232 = Not Equal To 0?(x=w381) -> (x != 0?=w383:bool)
                      n233 = And(x=w383, y=w382) -> (x .and. y?=w377:bool)
                      n234 = Select(t=cluster{u32, u32}[] [{12369084, 12369084}, {6618880, 6618880}] ("Colors [4]"), s=w377, f=cluster{u32, u32}[] [{12369084, 12369084}, {12369084, 12369084}] ("Colors [4]")) -> (s? t:f=w378:cluster{u32, u32}[])
                      n235 = property on="Align 2" class="Bool (strict)"("Colors [4]"=w378) -> ()  [unwired: 2 in, 2 out]
                    }
                    frame "?PHLDP" {
                      n236 = Decimal String To Number(string=w384) -> (number=w385:i32)  [unwired: 2 in, 1 out]
                      n237 = Not Equal To 0?(x=w385) -> (x != 0?=w388:bool)
                      n238 = local read "Dither hold"() -> (w386:bool)
                      n239 = And(x=w388, y=w386) -> (x .and. y?=w387:bool)
                      n240 = case shown="False" w387 {
                        frame False {
                          n241 = property on="Dither hold" class="Bool (strict)"("Colors [4]"=cluster{u32, u32}[] [{12369084, 12369084}, {12369084, 12369084}]) -> ()  [unwired: 2 in, 2 out]
                        }
                        frame True {
                          n242 = property on="Dither hold" class="Bool (strict)"("Colors [4]"=cluster{u32, u32}[] [{12369084, 12369084}, {6618880, 6618880}]) -> ()  [unwired: 2 in, 2 out]
                        }
                      }
                    }
                    frame "?UF" {
                      n243 = Decimal String To Number(string=w393) -> (number=w392:i32)  [unwired: 2 in, 1 out]
                      n244 = Round To Nearest(number=w392) -> (nearest integer value=→"Power (mW)":i32)
                    }
                    frame "?PFIXED" {
                      n245 = Decimal String To Number(string=w396) -> (number=w395:i32)  [unwired: 2 in, 1 out]
                      n246 = Round To Nearest(number=w395) -> (nearest integer value=→"Power 2":i32)
                    }
                    frame "?GDD" {
                      n247 = Decimal String To Number(string=w398) -> (number=w397:i32)  [unwired: 2 in, 1 out]
                      n248 = property on="GDD" class="DigNum (strict)"("Value"=w397) -> ()  [unwired: 2 in, 2 out]
                      n249 = shared-variable "My Computer\\Laser Library.lvlib\\GDD"(w397) -> ()  [unwired: 1 in, 1 out]
                    }
                    frame "?GDDMAX" {
                      n250 = Decimal String To Number(string=w406) -> (number=w404:i32)  [unwired: 2 in, 1 out]
                      n251 = Divide(x=w404, y=1000.0) -> (x/y=w400:dbl)
                      n252 = Round To Nearest(number=w400) -> (nearest integer value=w399:dbl)
                      n253 = Number To Decimal String(number=w399) -> (decimal integer string=w403:string)  [unwired: 1 in]
                      n254 = Concatenate Strings(w403, "k" ("string")) -> (→"Max":string)
                    }
                    frame "?TS" {
                      n255 = Decimal String To Number(string=w408) -> (number=→"Tunning Status":i32)  [unwired: 2 in, 1 out]
                    }
                    frame "?MDLK" {
                      n256 = Decimal String To Number(string=w410) -> (number=w411:i32)  [unwired: 2 in, 1 out]
                      n257 = Not Equal To 0?(x=w411) -> (x != 0?=→"ModeLocked":bool)
                    }
                    frame "?ST" {
                      "Operating Status" <- w412
                    }
                    frame "?F" {
                      "Faults" <- w413
                    }
                    frame "?RH" {
                      n258 = Decimal String To Number(string=w424) -> (number=w423:i32)  [unwired: 2 in, 1 out]
                      n259 = local read "Humidity Threshold"() -> (w414:dbl)
                      n260 = local read "Operating Status"() -> (w417:string)
                      n261 = local read "Laser Info"() -> (w420:i32)
                      n262 = Concatenate Strings(w417, "\nHigh Humidity") -> (w415:string)
                      n263 = Greater?(x=w423, y=w414) -> (0:w422:bool)
                      n264 = Select(t=w415, s=w422, f=w417) -> (s? t:f=w418:string)
                      n265 = Select(t=2, s=w422, f=w420) -> (s? t:f=w421:i32)
                      n266 = local write "Operating Status"(w418) -> ()
                      n267 = local write "Laser Info"(w421) -> ()
                    }
                    frame "?BT" {
                      n268 = Decimal String To Number(string=w426) -> (number=→"Baseplate Temp (C)":i32)  [unwired: 2 in, 1 out]
                    }
                  }
                }
                n269 = Decimal String To Number(string=w314) -> (number=w315:i32)  [unwired: 2 in, 1 out]
                n270 = local read "Operating Status"() -> (w316:string)
                n271 = Equal To 0?(x=w315) -> (x = 0?=w313:bool)
                n272 = Select(t=w316, s=w313, f=w314) -> (s? t:f=w317:string)
                n273 = Initialize Array(w317, 4 ("dimension size")) -> (w318:string[])
                n274 = property on="Laser Status" class="Bool (strict)"("Strings [4]"=w318) -> ()  [unwired: 2 in, 2 out]
              }
              frame #2 {
                n275 = local read "Tunning Status"() -> (w431:i32)
                n276 = local read "Laser Info"() -> (w429:i32)
                n277 = Equal To 0?(x=w431) -> (x = 0?=w432:bool)
                n278 = Not Equal To 0?(x=w429) -> (x != 0?=w428:bool)
                n279 = And(x=w432, y=w428) -> (x .and. y?=w430:bool)
                n280 = Equal?(x=w429, y=2.0) -> (x = y?=w434:bool)
                n281 = case shown="False" w434 {
                  tunnel: w430 -> [w436 _]
                  tunnel: [w435 cluster{u32, u32}[] [{16723218, 15670016}, {16721170, 16725034}] ("Colors [4]")] -> w427
                  frame False {
                    n282 = case shown="True" w436 {
                      tunnel: [cluster{u32, u32}[] [{10682272, 10682272}, {12451729, 12451729}] ("Colors [4]") w439] -> w435
                      frame False {
                        w438 = FALSE
                        n283 = local write "Laser Control"(w438) -> ()
                        "Laser Status" <- w438
                      }
                      frame True {
                        w444 = TRUE ("Laser Status")
                        n284 = local read "Operating Status"() -> (w443:string)
                        n285 = local write "Laser Control"(w444) -> ()
                        n286 = local write "Laser Status"(w444) -> ()
                        n287 = Equal?(x=w443, y="OK") -> (x = y?=w440:bool)
                        n288 = Select(t=cluster{u32, u32}[] [{6618880, 6618880}] ("Colors [4]"), s=w440, f=cluster{u32, u32}[] [{16762130, 16762130}, {10441728, 10441728}, {10441728, 10441728}] ("Colors [4]")) -> (s? t:f=w439:cluster{u32, u32}[])
                      }
                    }
                  }
                  frame True {
                  }
                }
                n289 = property on="Laser Status" class="Bool (strict)"("Colors [4]"=w427) -> ()  [unwired: 2 in, 2 out]
              }
              frame #3 {
                w450 = 2.0 ("y")
                w453 = 30
                n290 = Array Size(array=w448) -> (size(s)=w464:i32[])
                n291 = Index Array(array=w464, index=0) -> (element=w461:i32)
                n292 = Index Array(array=w464, index=1) -> (element=w460:i32)
                n293 = Multiply(x=w461, y=w460) -> (x*y=w458:i32)
                n294 = Divide(x=w458, y=w453) -> (x/y=w459:dbl)
                n295 = Divide(x=w453, y=w450) -> (x/y=w454:dbl)
                n296 = Reshape Array(w448, w458) -> (w457:string[])
                n297 = Subtract(x=w450, y=2.0) -> (x-y=w451:dbl)
                n298 = Round Toward +Infinity(x=w459) -> (ceil(x): smallest int >= x=w452:dbl)
                n299 = Initialize Array("", w454, w451) -> (w455:string[][])
                n300 = for {
                  N: w452 -> [_]
                  tunnel: w453 -> [w478]
                  shift-right: [w476] -> _
                  shift-left: w457 -> [w477]
                  tunnel: w453 -> [w472]
                  tunnel: w450 -> [w465]
                  shift-right: [w466] -> w447
                  shift-left: w455 -> [w468]
                  i -> [w475]
                  n301 = Divide(x=w472, y=w465) -> (x/y=w471:dbl)
                  n302 = Multiply(x=w475, y=w465) -> (x*y=w467:dbl)
                  n303 = Round Toward -Infinity(1:w471) -> (0:w470:dbl)
                  n304 = Split 1D Array(array=w477, index=w478) -> (first subarray=w474:string[], second subarray=w476:string[])
                  n305 = Reshape Array(w474, w470, 2 ("dimension size")) -> (w469:string[][])
                  n306 = Insert Into Array(array=w468, index (col)=w467, new element=w469) -> (w466:string[][])  [unwired: 1 in]
                }
                "Query List" <- w447
              }
              frame #4 {
                n307 = shared-variable ".\\Laser Library.lvlib\\Remote WV"() -> (w479:dbl)  [unwired: 1 in, 1 out]
                n308 = feedback-in #2(w479) -> ()
                n309 = feedback #2(w479) -> (w481:dbl)
                n310 = Not Equal?(x=w479, y=w481) -> (x != y?=w480:bool)
                n311 = case shown="True" w480 {
                  tunnel: w479 -> [_ w482]
                  frame False {
                  }
                  frame True {
                    n312 = property on="Wavelength" class="DigNum (strict)"("Val(Sgnl)"=w482) -> ()  [unwired: 2 in, 2 out]
                  }
                }
              }
            }
            n313 = local read "State next step"() -> (w304:string)
            "queue #" <- w303
          }
          frame "Walker" {
            w489 = dbl[] [680.0, 730.0, 780.0, 830.0, 880.0, 930.0, 980.0, 1030.0, 980.0, 930.0, 880.0, 830.0, 780.0, 730.0, 680.0, 800.0] ("Array")
            n314 = Wait (ms)(milliseconds to wait=2000) -> ()  [unwired: 1 out]
            n315 = local read "Step"() -> (w491:dbl)
            n316 = Index Array(array=w489, index=w491) -> (element=w485:dbl)
            n317 = Array Size(array=w489) -> (size(s)=w488:i32)
            n318 = Increment(x=w491) -> (x+1=w487:dbl)
            n319 = property on="Wavelength" class="DigNum (strict)"("Val(Sgnl)"=w485) -> ()  [unwired: 2 in, 2 out]
            n320 = Equal?(x=w487, y=w488) -> (x = y?=w486:bool)
            n321 = case shown="True" w486 {
              tunnel: w487 -> [w494 _]
              tunnel: [TRUE FALSE ("Walking")] -> w484
              frame False {
                n322 = local write "Step"(w494) -> ()
              }
              frame True {
                n323 = local write "WV Walk"(FALSE) -> ()
                n324 = local write "State next step"("Writer") -> ()
              }
            }
            "Walking" <- w484
          }
          frame "Backuper" {
            n325 = local read "Backuper state"() -> (w499:string)
            n326 = case shown="\"BackupFinal\"" w499 {
              tunnel: w501 -> [_ w524]
              frame "BackupInit", Default {
                n327 = flat-sequence {
                  frame #0 {
                    n328 = Wait (ms)(milliseconds to wait=u32 30000) -> ()  [unwired: 1 out]
                    n329 = local write "Backuper state"("BackupFinal") -> ()
                  }
                  frame #1 {
                    n330 = local write "Refresh"(TRUE ("Refresh")) -> ()
                  }
                }
              }
              frame "BackupFinal" {
                n331 = local write "Backup"(FALSE ("Backup")) -> ()
                n332 = local write "State next step"("Writer") -> ()
                n333 = local write "Backuper state"("BackupInit") -> ()
                n334 = String To IP() -> (0:w518:u32)  [unwired: 1 in]
                n335 = local read "SavePath"() -> (w505:path)
                n336 = IP To String(2:w518) -> (0:w506:string)  [unwired: 1 in]
                n337 = call "create unique folder.vi"("string"=w506, "path 2"=w505) -> ("path"=w511:path)  [unwired: 9 in]
                n338 = Get Date/Time In Seconds() -> (seconds since 1Jan1904=w520:timestamp)
                n339 = Format Date/Time String(time format string (%c)="%Y-%m-%d-%H-%M-%S", seconds (now)=w520) -> (date/time string=w515:string)  [unwired: 1 in]
                n340 = Path To String(path=w511) -> (string=w517:string)
                n341 = Concatenate Strings(w517, "\\" ("string"), w515, ".csv" ("string")) -> (w514:string)
                n342 = String To Path(string=w514) -> (path=w513:path)
                n343 = call-poly <vilib>:"Write To Spreadsheet File.vi"("delimiter (\\t)"="," ("delimiter (\\t)"), "format (%s)"="%.6f" ("format (%.3f)"), "append to file? (new file:F)"=FALSE, "2D data"=w524, "file path (dialog if empty)"=w513) -> ()  [unwired: 2 in, 2 out]
                "Backing up" <- FALSE ("Backing up ...")
              }
            }
          }
          frame "Quiter" {
            n344 = Equal To 0?(x=w529) -> (x = 0?=w528:bool)
            n345 = case shown="True" w528 {
              tunnel: ["Quiter" "Writer"] -> w527
              tunnel: [FALSE w533] -> w526
              frame False {
              }
              frame True {
                n346 = local read "Sleep"() -> (w532:bool)
                n347 = case shown="True" w532 {
                  tunnel: [w536 _] -> w533
                  frame False {
                    n348 = local read "QUIT"() -> (w535:bool)
                    n349 = case shown="True" w535 {
                      tunnel: [_ w537] -> w536
                      frame False {
                      }
                      frame True {
                        w537 = TRUE
                        n350 = local write "QUIT"(FALSE) -> ()
                        n351 = local write "stop"(w537) -> ()
                      }
                    }
                  }
                  frame True {
                    w540 = FALSE ("Sleep")
                    n352 = Wait (ms)(milliseconds to wait=u32 5000) -> ()  [unwired: 1 out]
                    n353 = local write "State next step"("Writer" ("State next step")) -> ()
                    n354 = local write "Sleep"(w540) -> ()
                    n355 = local write "Sleeping"(w540) -> ()
                    n356 = property on="Laser Control" class="Bool (strict)"("Val(Sgnl)"=w540) -> ()  [unwired: 2 in, 2 out]
                  }
                }
              }
            }
          }
        }
      }
      n357 = while {
        tunnel: w50 -> [w61]
        tunnel: w49 -> [w57]
        tunnel: w48 -> [w53]
        tunnel: [w56] -> w47
        tunnel: [w55] -> w46
        stop <- "stop" stop-if-true
        n358 = Get Queue Status(queue=w61, error in (no error)=w53) -> (queue out=w58:refnum<queue>, error out=w54:errorcluster, # elements in queue=w60:i32)  [unwired: 1 in, 5 out]
        n359 = Not Equal To 0?(x=w60) -> (x != 0?=w59:bool)
        n360 = case shown="True" w59 {
          tunnel: w58 -> [_ w76]
          tunnel: w57 -> [w63 w71]
          tunnel: [w63 w68] -> w56
          tunnel: [w64 w67] -> w55
          tunnel: w54 -> [w64 w66]
          frame False {
          }
          frame True {
            n361 = local read "Command Line"() -> (w73:string)
            n362 = local read "Query backup List"() -> (w75:string[][])
            n363 = Dequeue Element(queue=w76, error in (no error)=w66) -> (element=w70:string, error out=w65:errorcluster)  [unwired: 1 in, 2 out]
            n364 = Equal?(x=w73, y=w70) -> (x = y?=w72:bool)
            n365 = call-dynamic "WriteRead.vi"("error in (no error)"=w65, "Command"=w70, "Serial in"=w71) -> ("error out"=w67:errorcluster, "Response"=w69:string, "Serial out"=w68:refnum<class "Serial.lvclass">)  [unwired: 6 in]
            n366 = case shown="True" w72 {
              tunnel: w69 -> [_ w81]
              frame False {
              }
              frame True {
                "Laser Response" <- w81
              }
            }
            n367 = Index Array(array=w75, index (col)=0 ("index (row)")) -> (element=w79:string[])  [unwired: 1 in]
            n368 = Search 1D Array(1D array=w79, element=w70) -> (index of element=w77:i32)  [unwired: 1 in]
            n369 = Replace Array Subset(array=w75, new element=w69, index (row)=w77, index (col)=1 ("disabled index (col)")) -> (w74:string[][])
            n370 = local write "Query backup List"(w74) -> ()
          }
        }
      }
      n371 = call-dynamic "Close.vi"("error in (no error)"=w46, "Serial in"=w47) -> ("error out"=w45:errorcluster)  [unwired: 8 in, 1 out]
      n372 = call <vilib>:"Simple Error Handler.vi"("error in (no error)"=w45) -> ()  [unwired: 1 in, 8 out]
    }
  }
